vi "CalcDesiredAttitude_SpaceMouse_Input.vi"(9 "Attitude_Increase_Speed":dbl=0.01 format="%#_13g", 10 "Old desired Attitude":T2, 11 "SpaceMouse_FilteredInput":T3) -> (2 "New desired Attitude":T1)   [LabVIEW 2013]
uses:
  Controls/SpaceMouse_FilteredInput.ctl
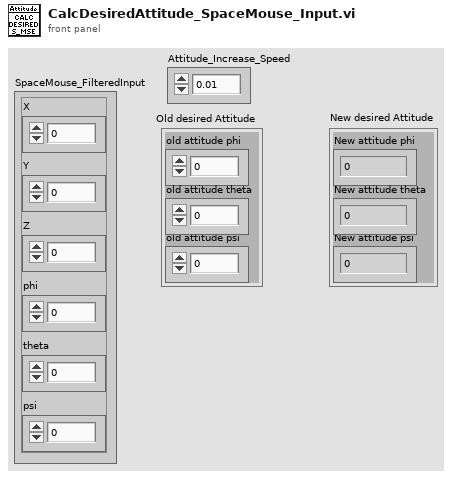
[diagram p1: front panel]
types:
  T1 = cluster{"New attitude phi":dbl, "New attitude theta":dbl, "New attitude psi":dbl}
  T2 = cluster{"old attitude phi":dbl, "old attitude theta":dbl, "old attitude psi":dbl}
  T3 = typedef "SpaceMouse_FilteredInput.ctl" = cluster{"X":dbl, "Y":dbl, "Z":dbl, "phi":dbl, "theta":dbl, "psi":dbl}
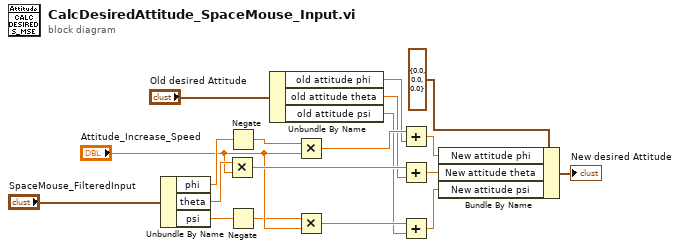
[diagram p0: block diagram]
diagram:
  n1 = Unbundle By Name("SpaceMouse_FilteredInput") -> ("phi"=w18:dbl, "theta"=w13:dbl, "psi"=w10:dbl)
  n2 = Multiply(x=w13, y="Attitude_Increase_Speed") -> (x*y=w14:dbl)
  n3 = Negate(x=w18) -> (-x=w2:dbl)
  n4 = Negate(x=w10) -> (-x=w1:dbl)
  n5 = Unbundle By Name("Old desired Attitude") -> ("old attitude phi"=w15:dbl, "old attitude theta"=w12:dbl, "old attitude psi"=w9:dbl)
  n6 = Multiply(x=w2, y="Attitude_Increase_Speed") -> (x*y=w19:dbl)
  n7 = Multiply(x=w1, y="Attitude_Increase_Speed") -> (x*y=w11:dbl)
  n8 = Add(x=w19, y=w15) -> (x+y=w5:dbl)
  n9 = Add(x=w14, y=w12) -> (x+y=w4:dbl)
  n10 = Add(x=w11, y=w9) -> (x+y=w3:dbl)
  n11 = Bundle By Name(cluster=T1 {"New attitude phi"=0.0, "New attitude theta"=0.0, "New attitude psi"=0.0} ("New Attitude"), "New attitude phi"=w5, "New attitude theta"=w4, "New attitude psi"=w3) -> (→"New desired Attitude":T1)
